vi "Save to AVI.vi"(6 "Enable saving":bool, 8 "error in (no error)":errorcluster, 10 "Refnum in":T2, 11 "AVI Refnum":T1) -> (0 "error out":errorcluster, 2 "Refnum out":T2, 3 "AVI Refnum (duplicate)":T1)   [LabVIEW 2020]
uses:
  <vilib>/vision/Image Controls.llb/IMAQ Image.ctl
  <vilib>/vision/Avi.llb/IMAQ AVI2 Refnum.ctl
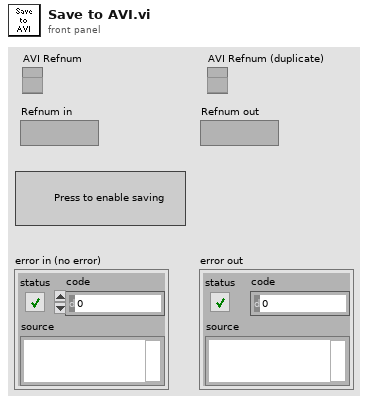
[diagram p1: front panel]
types:
  T1 = typedef "IMAQ AVI2 Refnum.ctl" = refnum<k20>
  T2 = typedef "IMAQ Image.ctl" = refnum<image>
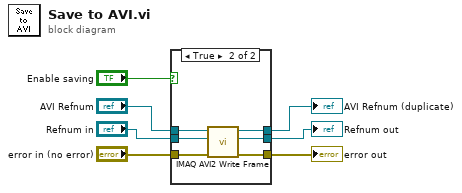
[diagram p0: block diagram]
diagram:
  n1 = case shown="True" "Enable saving" {
    tunnel: "AVI Refnum" -> [w10 w16]
    tunnel: "error in (no error)" -> [w8 w15]
    tunnel: [w10 w14] -> w6
    tunnel: [w8 w13] -> w7
    tunnel: "Refnum in" -> [w9 w12]
    tunnel: [w9 w11] -> w1
    frame False {
    }
    frame True {
      n2 = call "IMAQ AVI2 Write Frame"("error in (no error)"=w15, "Image"=w12, "AVI Refnum"=w16) -> ("error out"=w13:errorcluster, "Image Out (duplicate)"=w11:T2, "AVI Refnum (duplicate)"=w14:T1)  [unwired: 6 in]
    }
  }
  "Refnum out" <- w1
  "error out" <- w7
  "AVI Refnum (duplicate)" <- w6
